vi "Logistic Inverse CDF.vi"(9 "b":dbl=1.0, 10 "a":dbl, 11 "cdf(x)":dbl=0.1) -> (0 "error":i32, 3 "x":dbl=-2.1972245773362196)   [LabVIEW 2018, in "NI_Gmath.lvlib"]
doc: "Computes the continuous inverse cumulative distribution function (CDF) of the various distributions. You must manually select the polymorphic instance to use."
uses:
  NI_Gmath.lvlib
  st_error_code.ctl
panel:
  # "Logistic Inverse CDF"
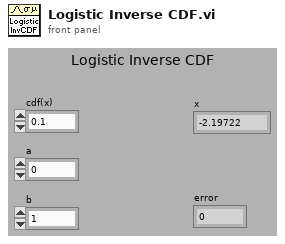
[diagram p1: front panel]
types:
  T1 = typedef "NI_Gmath.lvlib/st_error_code.ctl" = i32
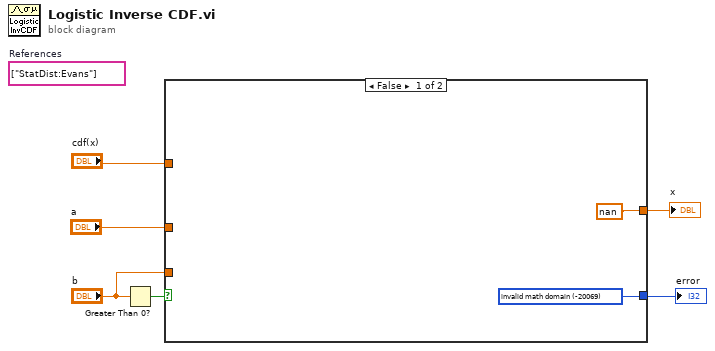
[diagram p0: block diagram]
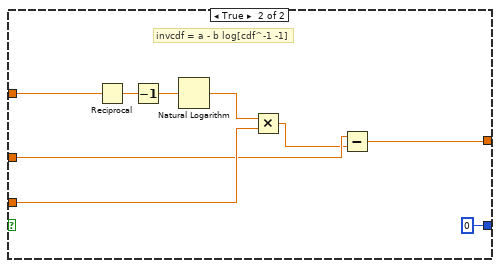
[diagram p2: hidden frame]
diagram:
  (unwired) string[] ["StatDist:Evans"]  # References
  n1 = Greater Than 0?(x="b") -> (x > 0?=w1:bool)
  n2 = case shown="False" w1 {
    tunnel: "b" -> [_ w13]
    tunnel: [w7 0 ("invalid math domain")] -> w2
    tunnel: [nan w10] -> w3
    tunnel: "cdf(x)" -> [_ w16]
    tunnel: "a" -> [_ w11]
    frame False {
      w7 = T1 -20069 items=["invalid math domain"=-20069, "Fourier interpolation size m >= n"=-20070, "empty array"=-20003] ("stat interp error code")
    }
    frame True {
      # "invcdf = a - b log[cdf^-1 -1]"
      n3 = Reciprocal(x=w16) -> (1/x=w15:dbl)
      n4 = Decrement(x=w15) -> (x-1=w14:dbl)
      n5 = Natural Logarithm(1:w14) -> (0:w12:dbl)
      n6 = Multiply(x=w12, y=w13) -> (x*y=w9:dbl)
      n7 = Subtract(x=w11, y=w9) -> (x-y=w10:dbl)
    }
  }
  "x" <- w3
  "error" <- w2
